vi "DriveGetLeftDist.vi"() -> (0 "Right dist":dbl, 1 "Left dist":dbl)   [LabVIEW 2020]
doc: "Gets left and right distance variables for drive"
uses:
  DriveGlobal.vi
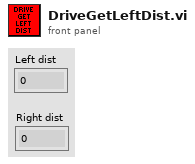
[diagram p1: front panel]
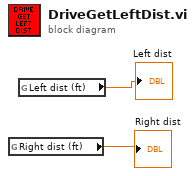
[diagram p0: block diagram]
diagram:
  n1 = global read "DriveGlobal.vi" "Right dist (ft)"() -> (→"Right dist":dbl)
  n2 = global read "DriveGlobal.vi" "Left dist (ft)"() -> (→"Left dist":dbl)
